vi "capturing_data.vi"() -> ()   [LabVIEW 2011]
panel:
  out "Salida Sub-Vi Backward":dbl(graph)=0.4127624224645584
  in  "b1":dbl=369.1752020780328
  in  "a0":dbl=579.8966661553599
  in  "a1":dbl=107.4314142898422
  in  "a2":dbl=14.57958812151553
  out "periodo de muestreo (ms)":dbl=33.333333333333336
  out "# Muestras":dbl=300.0
  in  "Frecuencia de generador":dbl=0.1
  in  "Frecuencia de muestreo":dbl=30.0
  out "Grafica General":dynamicdata(graph)=[{"t0"=timestamp(3466709157.666048 s since 1904-01-01), "dt"=1.0, "Y"=[0.4127624224645584]}, {"t0"=timestamp(3466709157.6760488 s since 1904-01-01), "dt"=1.0, "Y"=[0.4136778394660711]}, {"t0"=timestamp(3466709157.6760488 s since 1904-01-01), "dt"=1.0, "Y"=[0.4854053593120564]}]
  out "i":i32=299
  in  "A":dbl=1.0
  in  "tf":dbl=5.0
  in  "t0":dbl
  in  "Ring":u16(ring)=1 items=["step"=1, "gate"=2, "rampa"=3, "seno"=4]
  out "Señal sensada":dbl(graph)=0.48424496688060725
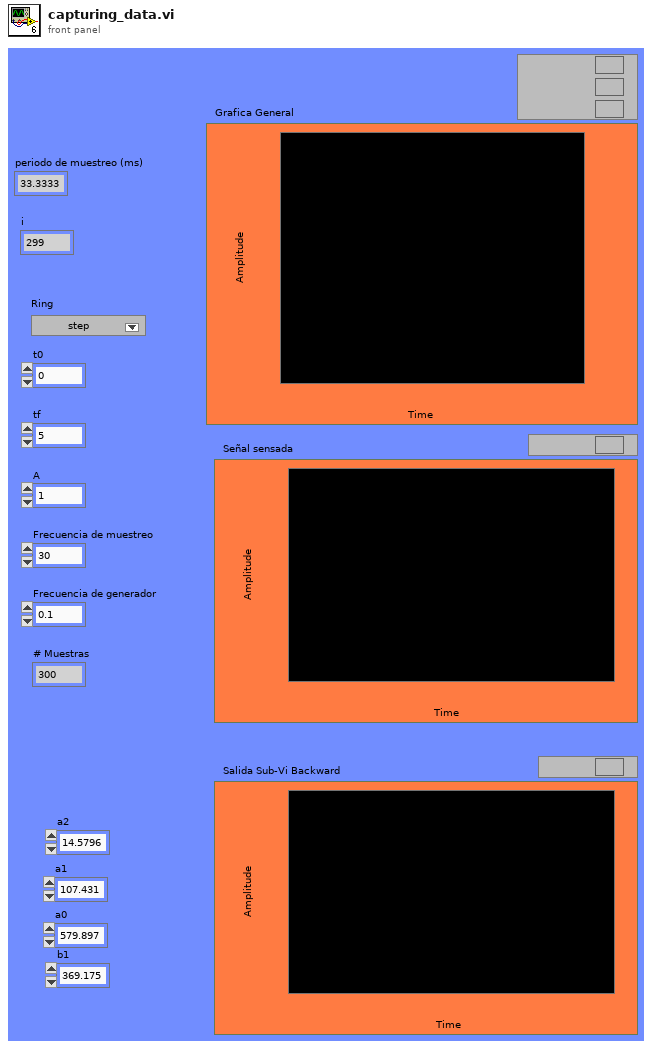
[diagram p1: front panel]
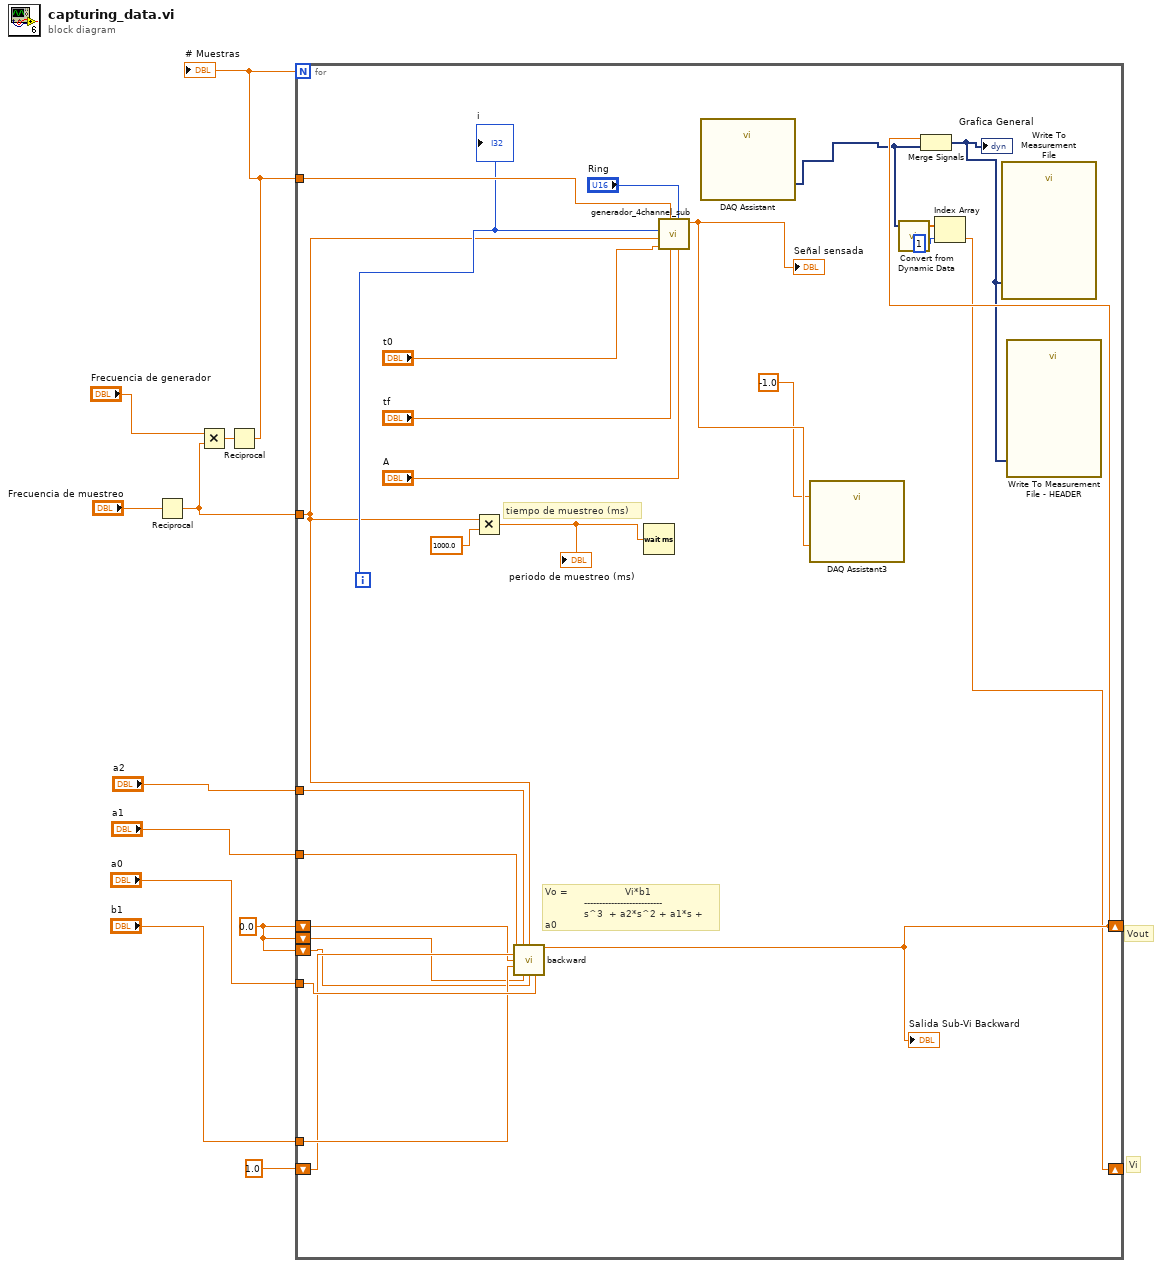
[diagram p0: block diagram]
diagram:
  w1 = 0.0
  # "Vout"
  # "Vi"
  n1 = Reciprocal(x="Frecuencia de muestreo") -> (1/x=w9:dbl)
  n2 = Multiply(x="Frecuencia de generador", y=w9) -> (x*y=w8:dbl)
  n3 = Reciprocal(x=w8) -> (1/x=w7:dbl)
  "# Muestras" <- w7
  n4 = for {
    N: w7 -> [_]
    tunnel: w7 -> [w32]
    tunnel: w9 -> [w26]
    tunnel: "a2" -> [w28]
    tunnel: "a1" -> [w27]
    tunnel: "a0" -> [w25]
    tunnel: "b1" -> [w24]
    shift-right: [w23] -> _
    shift-left: w1 -> [w20]
    shift-left: w1 -> [w19]
    shift-left: w1 -> [w18]
    shift-right: [w12] -> _
    shift-left: 1.0 -> [w21]
    i -> [w31]
    # "Vo =                   Vi*b1\n             --------------------------\n             s^3  + a2*s^2 + a1*s + a0"
    # "tiempo de muestreo (ms)"
    n5 = Multiply(x=w26, y=1000.0) -> (x*y=w29:dbl)
    "periodo de muestreo (ms)" <- w29
    n6 = call "backward.vi"("a1"=w27, "a2"=w28, "T"=w26, "Vi(n-1)"=w21, "Vo(n-1)"=w20, "b1"=w24, "Vo(n-2)"=w19, "Vo(n-3)"=w18, "a0"=w25) -> ("Vo (salida)"=w23:dbl)  [unwired: 6 in]
    "Salida Sub-Vi Backward" <- w23
    n7 = Wait (ms)(milliseconds to wait=w29) -> ()  [unwired: 1 out]
    n8 = call "generador_4channel_sub.vi"("A"="A", "Ring"="Ring", "t1"="tf", "N"=w32, "t0"="t0", "T"=w26, "i"=w31) -> ("Waveform Chart"=w15:dbl)  [unwired: 4 in]
    "Señal sensada" <- w15
    n9 = call "DAQ Assistant"() -> ("data"=w16:dynamicdata)  [unwired: 17 in, 2 out]
    n10 = call "DAQ Assistant3"("data"=w15, "timeout (s)"=-1.0) -> ()  [unwired: 16 in, 2 out]
    n11 = call "Convert from Dynamic Data"("Dynamic Data Type"=w16) -> ("Array"=w22:dbl[])  [unwired: 3 in]
    n12 = Merge Signals(w23, w16) -> (w17:dynamicdata)
    "Grafica General" <- w17
    n13 = Index Array(array=w22, index=1) -> (element=w12:dbl)
    n14 = call "Write To Measurement File"("Signals"=w17) -> ()  [unwired: 16 in, 3 out]
    n15 = call "Write To Measurement File - HEADER"("Signals"=w17) -> ()  [unwired: 16 in, 3 out]
    "i" <- w31
  }
